vi "Separate_Detections_into_Good_and_Bad.vi"(6 "Dataset":T2, 8 "error in":errorcluster, 10 "Pixel Scores":sgl[][][](array[numeric]), 11 "Image Scores":sgl[](array[numeric])) -> (0 "error out":errorcluster, 2 "Bad Samples":T1[](array[typedef]), 3 "Good Samples":T1[](array[typedef]))   [LabVIEW 2020]
uses:
  Controls/Detection_Results.ctl
  <vilib>/Ngene/DeepLTK Anomaly Detection Addon/Toolkit/API/Controls/NNPC_DS_Custom_Data.ctl
  <vilib>/Ngene/DeepLTK Anomaly Detection Addon/Toolkit/DeepLTK_Anomaly_Detection_Addon.lvlib
  <vilib>/Ngene/Deep Learning Toolkit/Toolkit/NN_Data/API/NN_Dims(C,H,W).ctl
  <vilib>/Ngene/Deep Learning Toolkit/Toolkit/Deep_Learning_Toolkit_by_Ngene.lvlib
  <vilib>/Ngene/Deep Learning Toolkit/Toolkit/NN_Data/Controls/DataRef_Types/4D/NN_Data_ref(4D_SGL).ctl
  <vilib>/Ngene/Deep Learning Toolkit/Toolkit/NN_Data/API/DataSet/DataSet_Types/NN_DataSet(In3D_Out3D).ctl
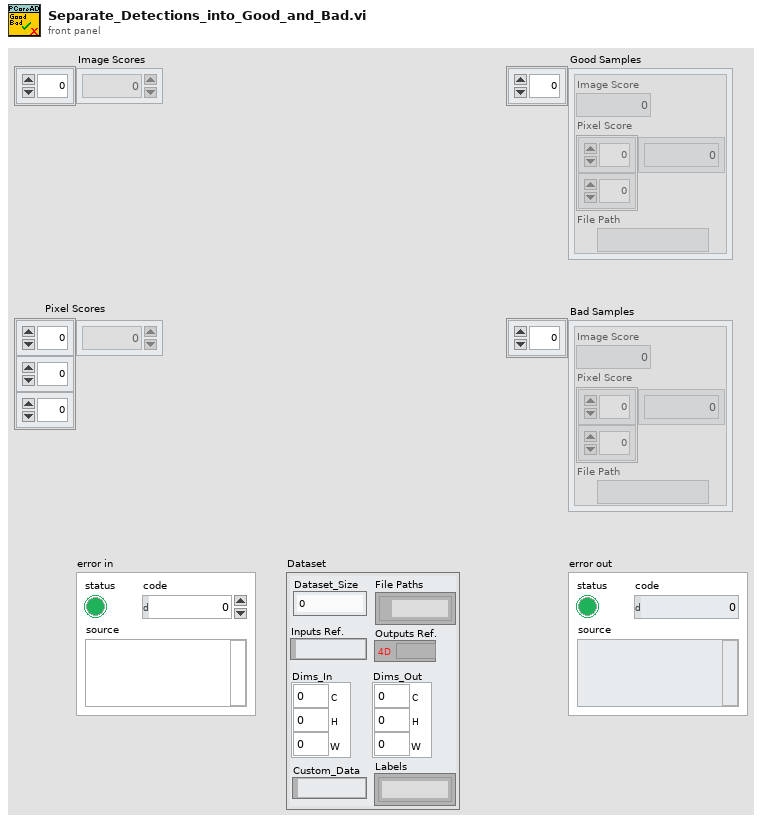
[diagram p1: front panel]
types:
  T1 = typedef "Detection_Results.ctl" = cluster{"Image Score":sgl, "Pixel Score":sgl[][], "File Path":path}
  T2 = typedef "Deep_Learning_Toolkit_by_Ngene.lvlib/NN_DataSet(In3D_Out3D).ctl" = cluster{"Dataset_Size":i32, "Dims_In":T3, "Labels":string[], "File Paths":path[], "Outputs Ref.":T4, "Inputs Ref.":variant, "Dims_Out":T3, "Custom_Data":variant}
  T3 = typedef "Deep_Learning_Toolkit_by_Ngene.lvlib/NN_Dims(C,H,W).ctl" = cluster{"C":i32, "H":i32, "W":i32}
  T4 = typedef "Deep_Learning_Toolkit_by_Ngene.lvlib/NN_Data_ref(4D_SGL).ctl" = refnum<data-value>
  T5 = typedef "DeepLTK_Anomaly_Detection_Addon.lvlib/NNPC_DS_Custom_Data.ctl" = cluster{"HasPixelGT?":bool, "ImageGT":refnum<data-value>, "PixelGT":refnum<data-value>}
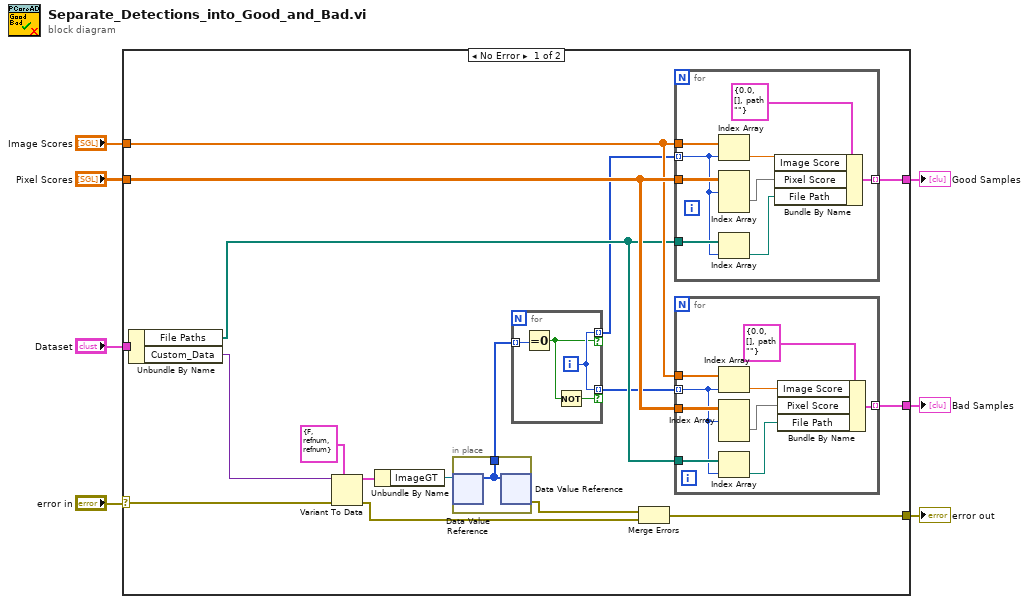
[diagram p0: block diagram]
diagram:
  n1 = case shown="No Error" "error in" {
    selector: "error in" -> [w15 w48]
    tunnel: [w24 w48] -> w5
    tunnel: "Image Scores" -> [w22 _]
    tunnel: "Pixel Scores" -> [w23 _]
    tunnel: "Dataset" -> [w21 _]
    tunnel: [w19 _] -> w3
    tunnel: [w18 _] -> w2
    frame No Error {
      n2 = Unbundle By Name(w21) -> ("File Paths"=w20:path[], "Custom_Data"=w16:variant)
      n3 = Variant To Data(error in=w15, type=T5 {"HasPixelGT?"=FALSE, "ImageGT"=refnum, "PixelGT"=refnum} ("DS_Custom_Data"), Variant=w16) -> (data=w17:T5, error out=w10:errorcluster)
      n4 = Unbundle By Name(w17) -> ("ImageGT"=w14:refnum<data-value>)
      n5 = in-place {
        in-place-border: [w38] -> w13
        n6 = in-place-dvr #1(w14) -> (w38:i32[])  [unwired: 1 out]
        n7 = in-place-dvr #1(w38) -> (w9:errorcluster)  [unwired: 1 out]
      }
      n8 = for {
        tunnel: [w37] -> w12 mode=indexing if=w35
        tunnel: [w37] -> w11 mode=indexing if=w34
        tunnel: w13 -> [w36] mode=indexing
        i -> [w37]
        n9 = Equal To 0?(x=w36) -> (x = 0?=w35:bool)
        n10 = Not(x=w35) -> (.not. x?=w34:bool)
      }
      n11 = Merge Errors(w9, w10) -> (w24:errorcluster)
      n12 = for {
        tunnel: w22 -> [w32]
        tunnel: w23 -> [w33]
        tunnel: w12 -> [w30] mode=indexing
        tunnel: w20 -> [w31]
        tunnel: [w27] -> w19 mode=indexing
        n13 = Index Array(array=w32, index=w30) -> (element=w29:sgl)
        n14 = Index Array(array=w33, index (dim 0)=w30) -> (element=w28:sgl[][])  [unwired: 2 in]
        n15 = Index Array(array=w31, index=w30) -> (element=w25:path)
        n16 = Bundle By Name(cluster=T1 {"Image Score"=0.0, "Pixel Score"=[], "File Path"=path ""}, "Image Score"=w29, "Pixel Score"=w28, "File Path"=w25) -> (w27:T1)
      }
      n17 = for {
        tunnel: w22 -> [w47]
        tunnel: w11 -> [w44] mode=indexing
        tunnel: w23 -> [w46]
        tunnel: w20 -> [w45]
        tunnel: [w41] -> w18 mode=indexing
        n18 = Index Array(array=w47, index=w44) -> (element=w43:sgl)
        n19 = Index Array(array=w46, index (dim 0)=w44) -> (element=w42:sgl[][])  [unwired: 2 in]
        n20 = Index Array(array=w45, index=w44) -> (element=w39:path)
        n21 = Bundle By Name(cluster=T1 {"Image Score"=0.0, "Pixel Score"=[], "File Path"=path ""}, "Image Score"=w43, "Pixel Score"=w42, "File Path"=w39) -> (w41:T1)
      }
    }
    frame Error {
    }
  }
  "error out" <- w5
  "Bad Samples" <- w2
  "Good Samples" <- w3
